vi "PowerLawFit.vi"(5 "MinFitZ":dbl, 7 "MaxFitZ":dbl, 8 "ZeroDisplacement?":enum16{"Allow d0", "No displacement"}(ring), 9 "Zref":dbl, 10 "U/Uref":dbl[](array[numeric]), 11 "z":dbl[](array[numeric])) -> (0 "PowerLaw":T2, 1 "PowerLawFitEquation":string, 2 "CroppedData":cluster{"X Out":dbl[], "Y Out":dbl[]}, 3 "FitCurve":T3)   [LabVIEW 2014]
uses:
  PowerLaw.ctl
  <vilib>/Analysis/6fits.llb/Curve Fitting Criteria.ctl
  <vilib>/Analysis/6fits.llb/Remove Outliers (Range).vi
  <vilib>/gmath/NumericalOptimization/Nonlinear Curve Fit LM formula string.vi
  <vilib>/gmath/NI_Gmath.lvlib
  <vilib>/Analysis/NI_AALPro.lvlib
panel:
  in  "noDisplacementmethod":T1=1 items=["Least Square", "Least Absolute Residual", "Bisquare"]
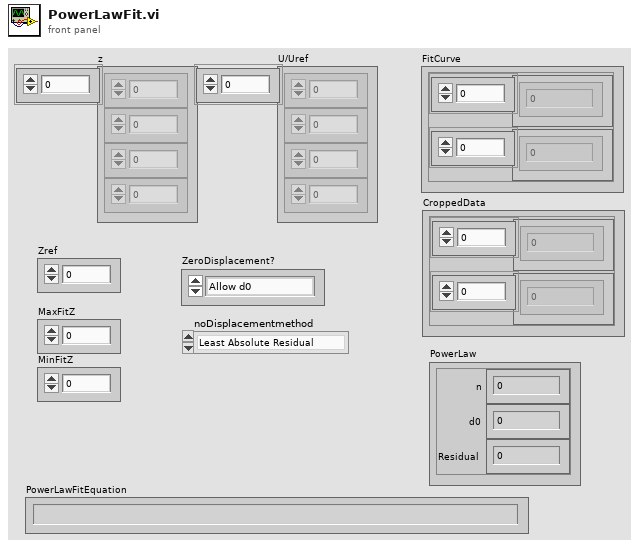
[diagram p1: front panel]
types:
  T1 = typedef "NI_AALPro.lvlib/Curve Fitting Criteria.ctl" = u16
  T2 = typedef "PowerLaw.ctl" = cluster{"n":dbl, "d0":dbl, "Residual":dbl}
  T3 = cluster{"Array":dbl[], "best nonlinear fit":dbl[]}
  T4 = cluster{"model":string, "Parameters":string[], "x":string}
  T5 = cluster{"amp min":dbl, "amp max":dbl, "power min":dbl, "power max":dbl, "offset min":dbl, "offset max":dbl}
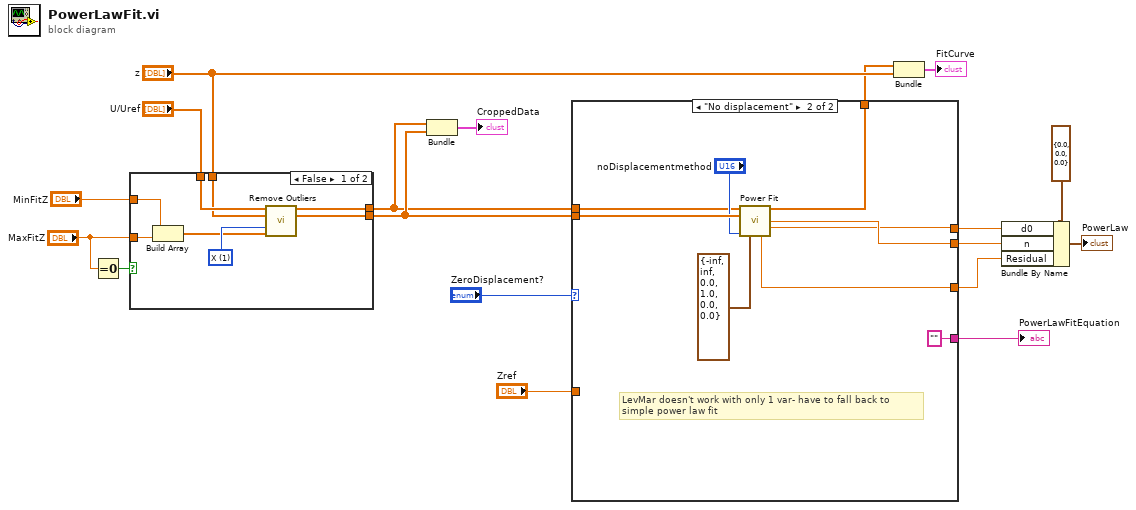
[diagram p0: block diagram]
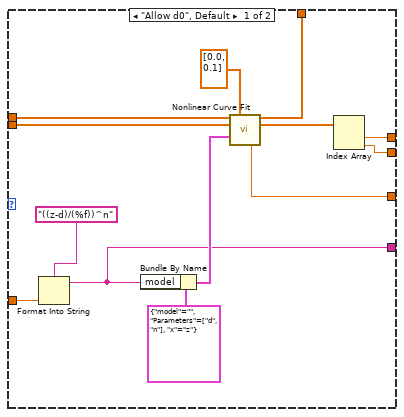
[diagram p2: hidden frame]
diagram:
  n1 = Equal To 0?(x="MaxFitZ") -> (x = 0?=w14:bool)
  n2 = case shown="False" w14 {
    tunnel: [w26 w27] -> w11
    tunnel: [w25 w28] -> w12
    tunnel: "U/Uref" -> [w23 w27]
    tunnel: "z" -> [w22 w28]
    tunnel: "MaxFitZ" -> [w20 _]
    tunnel: "MinFitZ" -> [w19 _]
    frame False {
      w24 = u16 1 items=["x", "X", "X and Y"] ("range type")
      n3 = Build Array(w19, w20) -> (w21:dbl[])
      n4 = call-poly <vilib>:"Remove Outliers.vi"("Y"=w23, "X"=w22, "range type"=w24, "Range"=w21) -> ("Y Out"=w26:dbl[], "X Out"=w25:dbl[])  [unwired: 7 in, 3 out]
    }
    frame True {
    }
  }
  n5 = Bundle("U/Uref"=w11, "z"=w12) -> (→"CroppedData":cluster{"U/Uref":dbl[], "z":dbl[]})  [unwired: 1 in]
  n6 = case shown="\"No displacement\"" "ZeroDisplacement?" {
    tunnel: [w39 ""] -> w13
    tunnel: w12 -> [w38 w45]
    tunnel: w11 -> [w37 w43]
    tunnel: [w36 w47] -> w7
    tunnel: [w35 w49] -> w6
    tunnel: "Zref" -> [w34 _]
    tunnel: [w33 w50] -> w9
    tunnel: [w29 w42] -> w3
    frame "Allow d0", Default {
      n7 = Format Into String(format string="((z-d)/(%f))^n" ("vonKarman Spectrum"), w34) -> (resulting string=w39:string)  [unwired: 2 in, 1 out]
      n8 = Bundle By Name(cluster=T4 {"model"="", "Parameters"=["d", "n"], "x"="z"} ("model description"), "model"=w39) -> (w41:T4)
      n9 = call-poly <vilib>:"Nonlinear Curve Fit.vi"("Y"=w37, "initial parameters"=dbl[] [0.0, 0.1], "X"=w38, "model description"=w41) -> ("best nonlinear fit"=w33:dbl[], "best fit parameters"=w40:dbl[], "residue"=w29:dbl)  [unwired: 7 in, 2 out]
      n10 = Index Array(array=w40) -> (element #1=w36:dbl, element #2=w35:dbl)  [unwired: 2 in]
    }
    frame "No displacement" {
      # "LevMar doesn't work with only 1 var- have to fall back to\nsimple power law fit"
      n11 = call <vilib>:"Power Fit.vi"("Y"=w43, "X"=w45, "method"="noDisplacementmethod", "parameter bounds"=T5 {"amp min"=-inf, "amp max"=inf, "power min"=0.0, "power max"=1.0, "offset min"=0.0, "offset max"=0.0}) -> ("Best Power Fit"=w50:dbl[], "power"=w49:dbl, "offset"=w47:dbl, "residue"=w42:dbl)  [unwired: 6 in, 2 out]
    }
  }
  "PowerLawFitEquation" <- w13
  n12 = Bundle("Best Power Fit"=w9, "z"="z") -> (→"FitCurve":cluster{"Best Power Fit":dbl[], "z":dbl[]})  [unwired: 1 in]
  n13 = Bundle By Name(cluster=cluster{"n":dbl, "d0":dbl, "Residual":dbl} {"n"=0.0, "d0"=0.0, "Residual"=0.0} ("PowerLaw"), "d0"=w7, "n"=w6, "Residual"=w3) -> (→"PowerLaw":cluster{"n":dbl, "d0":dbl, "Residual":dbl})
